vi "Read-Write-Signals.UpdateStateWithRef.vi"(0 "XRef":T13, 1 "Old State":T12, 2 "Version":T10) -> (14 "Is Good?":T9, 15 "Reply":T7, 17 "State Out":T1)   [LabVIEW 2015, in "Read-Write-Signals.xnode"]
uses:
  Read-Write-Signals.xnode
  <vilib>/XNodeSupport/XNodeXNodeRef.ctl
  <vilib>/XNodeSupport/XNodeVariant.ctl
  <vilib>/XNodeSupport/XNodeVersion.ctl
  <vilib>/XNodeSupport/XNodeUShort.ctl
  <vilib>/XNodeSupport/XNodeBool.ctl
  <vilib>/XNodeSupport/XNodeStringArray.ctl
  <vilib>/XNodeSupport/XNodeString.ctl
  State.ctl
  Read-Write-Signals Item.ctl
  Read-Write-Signals Sub Item.ctl
  Read-Write-Signals Sub Item Type.ctl
  Read-Write-Signals Selection.ctl
  Read-Write-Signals Display Selection.ctl
  <vilib>/XNodeSupport/NI_XNodeSupport.lvlib
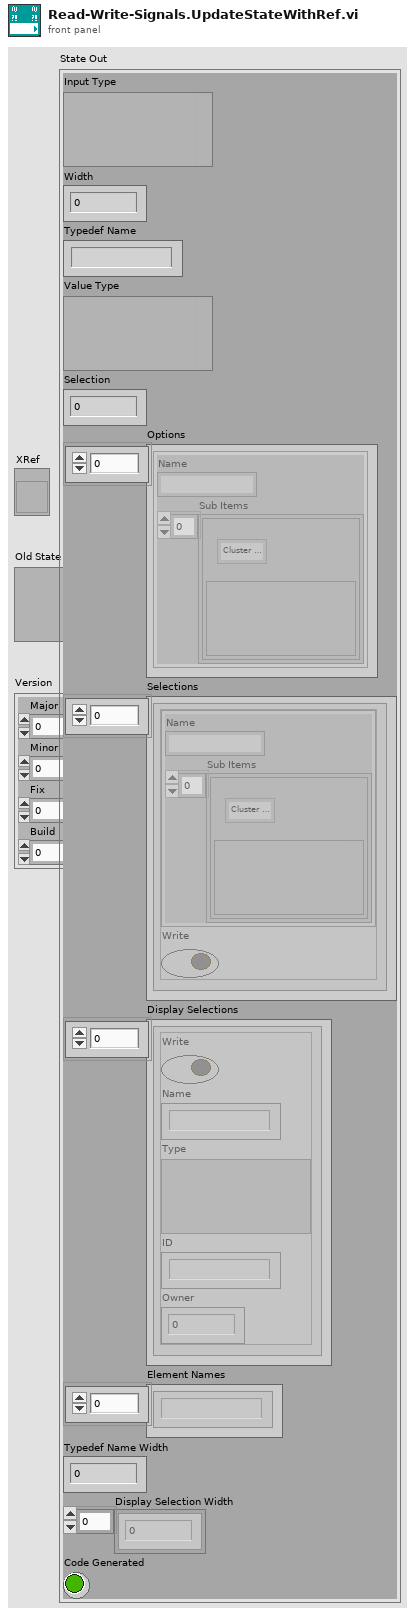
[diagram p1: front panel]
types:
  T1 = typedef "Read-Write-Signals.xnode/State.ctl" = cluster{"Input Type":variant, "Width":i32, "Typedef Name":string, "Value Type":variant, "Selection":i32, "Options":T2[], "Selections":T5[], "Display Selections":T6[], "Element Names":string[], "Typedef Name Width":i32, "Display Selection Width":i32[], "Code Generated":bool}
  T2 = typedef "Read-Write-Signals Item.ctl" = cluster{"Name":string, "Sub Items":T3[]}
  T3 = typedef "Read-Write-Signals Sub Item.ctl" = cluster{"Type":T4, "Value":variant}
  T4 = typedef "Read-Write-Signals Sub Item Type.ctl" = enum8{"Cluster Element", "Array Element", "Subarray"}
  T5 = typedef "Read-Write-Signals Selection.ctl" = cluster{"Item":T2, "Write":bool}
  T6 = typedef "Read-Write-Signals Display Selection.ctl" = cluster{"Write":bool, "Name":string, "Type":variant, "ID":string, "Owner":i32}
  T7 = typedef "NI_XNodeSupport.lvlib/XNodeStringArray.ctl" = T8[]
  T8 = typedef "NI_XNodeSupport.lvlib/XNodeString.ctl" = string
  T9 = typedef "NI_XNodeSupport.lvlib/XNodeBool.ctl" = bool
  T10 = typedef "NI_XNodeSupport.lvlib/XNodeVersion.ctl" = cluster{"Major":T11, "Minor":T11, "Fix":T11, "Build":T11}
  T11 = typedef "NI_XNodeSupport.lvlib/XNodeUShort.ctl" = u16
  T12 = typedef "NI_XNodeSupport.lvlib/XNodeVariant.ctl" = variant
  T13 = typedef "NI_XNodeSupport.lvlib/XNodeXNodeRef.ctl" = refnum<vi>
  T14 = cluster{"Input Type":variant, "Width":i32, "Typedef Name":string, "Value Type":variant, "Selection":i32, "Options":T2[], "Selections":T5[], "Display Selections":T6[], "Element Names":string[], "Typedef Name Width":i32, "Display Selection Width":i32[], "Code Generated":bool}
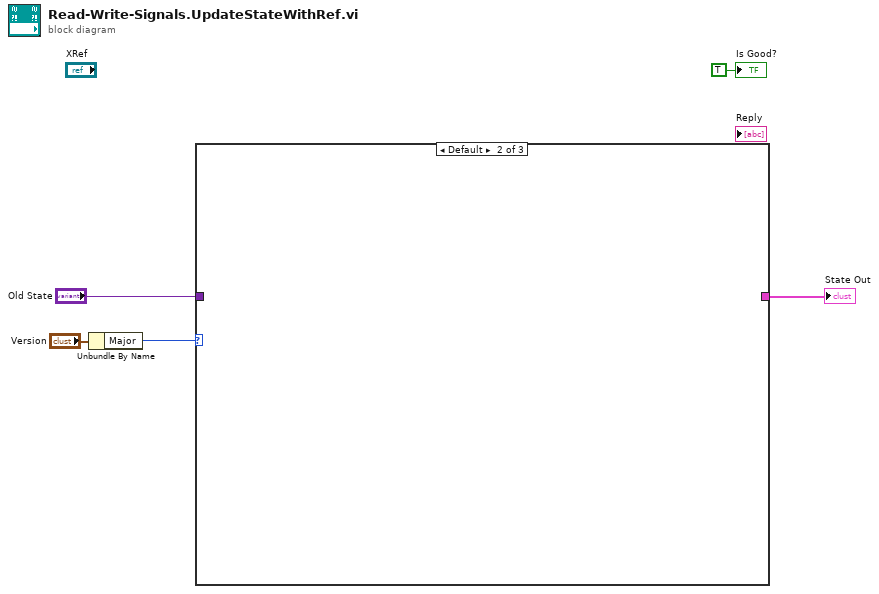
[diagram p0: block diagram]
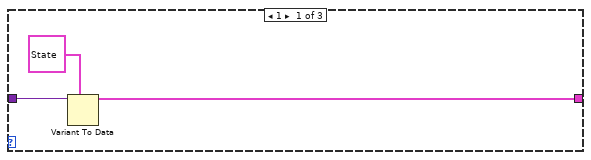
[diagram p2: hidden frame]
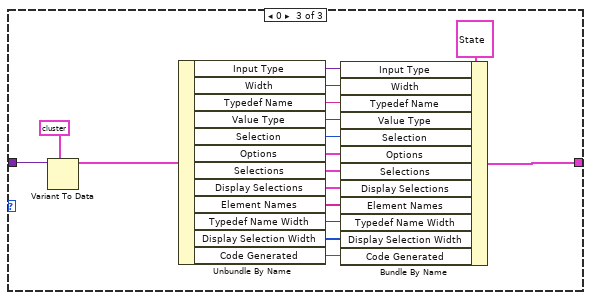
[diagram p3: hidden frame]
diagram:
  n1 = Unbundle By Name("Version") -> ("Major"=w3:T11)
  n2 = case shown="Default" w3 {
    tunnel: "Old State" -> [w8 _ w25]
    tunnel: [w6 _ w9] -> w2
    frame 1 {
      n3 = Variant To Data(type=T1 {"Input Type"=variant, "Width"=0, "Typedef Name"="", "Value Type"=variant, "Selection"=0, "Options"=[], "Selections"=[], "Display Selections"=[], "Element Names"=[], "Typedef Name Width"=0, "Display Selection Width"=[], "Code Generated"=FALSE} ("State Out"), Variant=w8) -> (data=w6:T1)  [unwired: 1 in, 1 out]
    }
    frame Default {
    }
    frame 0 {
      n4 = Variant To Data(type=T14 {"Input Type"=variant, "Width"=0, "Typedef Name"="", "Value Type"=variant, "Selection"=0, "Options"=[], "Selections"=[], "Display Selections"=[], "Element Names"=[], "Typedef Name Width"=0, "Display Selection Width"=[], "Code Generated"=FALSE} ("State Out"), Variant=w25) -> (data=w10:T14)  [unwired: 1 in, 1 out]
      n5 = Unbundle By Name(w10) -> ("Input Type"=w12:variant, "Width"=w13:i32, "Typedef Name"=w14:string, "Value Type"=w15:variant, "Selection"=w16:i32, "Options"=w17:T2[], "Selections"=w18:T5[], "Display Selections"=w19:T6[], "Element Names"=w20:string[], "Typedef Name Width"=w21:i32, "Display Selection Width"=w22:i32[], "Code Generated"=w23:bool)
      n6 = Bundle By Name(cluster=T1 {"Input Type"=variant, "Width"=0, "Typedef Name"="", "Value Type"=variant, "Selection"=0, "Options"=[], "Selections"=[], "Display Selections"=[], "Element Names"=[], "Typedef Name Width"=0, "Display Selection Width"=[], "Code Generated"=FALSE} ("State Out"), "Input Type"=w12, "Width"=w13, "Typedef Name"=w14, "Value Type"=w15, "Selection"=w16, "Options"=w17, "Selections"=w18, "Display Selections"=w19, "Element Names"=w20, "Typedef Name Width"=w21, "Display Selection Width"=w22, "Code Generated"=w23) -> (w9:T1)
    }
  }
  "State Out" <- w2
  "Is Good?" <- T9 TRUE ("Is Good?")
